vi "Find DMM classes.vi"(8 "error in (no error)":errorcluster, 11 "Files":path[](array[path])) -> (0 "error out":errorcluster, 2 "Class names":string[](array[string]), 3 "DMM classes":refnum<class "DMM.lvclass">[](array[class]))   [LabVIEW 2019, in "Configure Hardware.lvlib"]
uses:
  Configure Hardware.lvlib
  Common Components/Hardware/DMM/DMM.lvclass
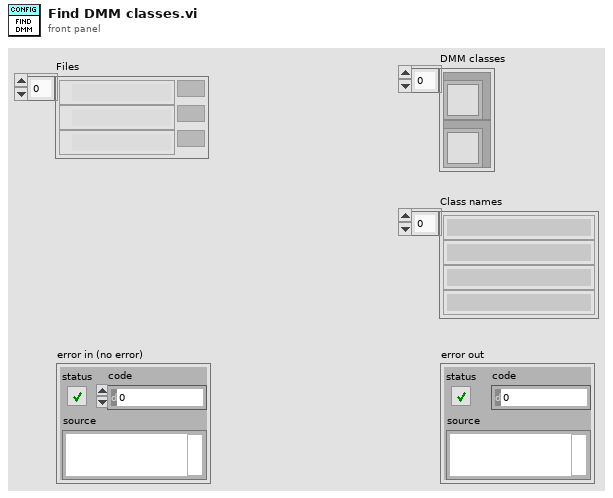
[diagram p1: front panel]
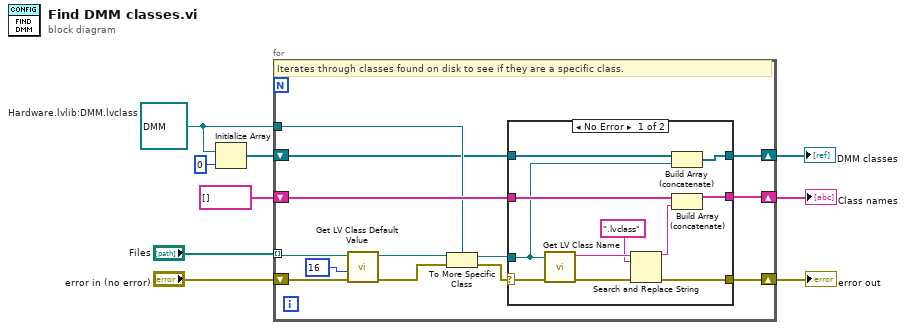
[diagram p0: block diagram]
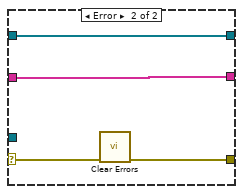
[diagram p2: hidden frame]
diagram:
  w4 = refnum<class "DMM.lvclass"> refnum  # Hardware.lvlib:DMM.lvclass
  n1 = Initialize Array(w4, 0 ("dimension size")) -> (w2:refnum<class "DMM.lvclass">[])
  n2 = for {
    tunnel: "Files" -> [w17] mode=indexing
    shift-right: [w12] -> w6
    shift-left: string[] [] -> [w19]
    shift-right: [w18] -> w9
    shift-left: "error in (no error)" -> [w20]
    tunnel: w4 -> [w15]
    shift-right: [w10] -> w1
    shift-left: w2 -> [w11]
    # "Iterates through classes found on disk to see if they are a specific class."
    n3 = call <vilib>:"Get LV Class Default Value.vi"("error in (no error)"=w20, "options"=u32 16, "class path"=w17) -> ("error out"=w21:errorcluster, "object"=w16:refnum<class>)  [unwired: 7 in]
    n4 = To More Specific Class(target class=w15, reference=w16, error in=w21) -> (specific class reference=w22:refnum<class "DMM.lvclass">, error out=w14:errorcluster)
    n5 = case shown="No Error" w14 {
      selector: w14 -> [w31 w36]
      tunnel: w22 -> [w24 _]
      tunnel: [w33 w37] -> w12
      tunnel: w19 -> [w32 w37]
      tunnel: [w29 w35] -> w18
      tunnel: w11 -> [w25 w34]
      tunnel: [w23 w34] -> w10
      frame No Error {
        n6 = call <vilib>:"Get LV Class Name.vi"("error in (no error)"=w31, "object"=w24) -> ("error out"=w30:errorcluster, "class name"=w28:string)  [unwired: 8 in]
        n7 = Search and Replace String(input string=w28, search string=".lvclass", error in=w30) -> (result string=w26:string, error out=w29:errorcluster)  [unwired: 5 in, 2 out]
        n8 = Build Array (concatenate)(w25, w24) -> (w23:refnum<class "DMM.lvclass">[])
        n9 = Build Array (concatenate)(w32, w26) -> (w33:string[])
      }
      frame Error {
        n10 = call <vilib>:"Clear Errors.vi"("error in (no error)"=w36) -> ("error out"=w35:errorcluster)  [unwired: 5 in, 1 out]
      }
    }
  }
  "error out" <- w9
  "Class names" <- w6
  "DMM classes" <- w1
